vi "Fit parameters chooser.vi"(0 "Stop signaller":refnum<class "Signaller.lvclass">, 5 "Fit parameters refnum":refnum<vi>, 7 "C refnum":refnum<vi>, 9 "Physical constants refnum":refnum<vi>, 11 "Simulation parameters semaphore":T1) -> ()   [LabVIEW 2015]
uses:
  Fit Parameters.ctl
  Physical Constants.ctl
  Motor controller/Signaller/Signaller.lvclass
  <vilib>/gmath/statdist.llb/Continuous PDF.vi
  <vilib>/gmath/statdist.llb/Normal PDF.vi
  <vilib>/gmath/NI_Gmath.lvlib
  <vilib>/Utility/config.llb/NI_LVConfig.lvlib
panel:
  in  "Overwrite selected preset":bool
  in  "Save as new preset":bool
  in  "Load from preset":bool
  in  "Choose preset":u16(ring) items=["Experimental data", "Test"]
  in  "Refresh graphs":bool
  in  "Update simulation parameters":bool
  in  "Physical constants":T2={"T1e (s)"=0.03, "T1n (s)"=1500.0}
  in  "C":dbl=0.000136073
  in  "Fit parameters":T3={"A"=0.572086, "S"=0.0835606, "M1"=140.286, "M2"=140.486}
  out "Steady state distribution":cluster{dbl[], dbl[]}(graph)
  out "Alpha/beta distributions":cluster{dbl[], dbl[]}[](graph)
  # "Explanation of fit parameters:\nThe parameters A, S, M1, and M2 control the distribution of alpha and beta as shown above. The steady state distribution will be computed from these.\nA: the height of the Gaussian distributions for alpha and beta\nS: the standard deviation of the Gaussian distributions for alpha and beta\nM1: the mean of the Gaussian distribution for beta\nM2: the mean of the Gaussian distribution for alpha"
  # "Internal controls"
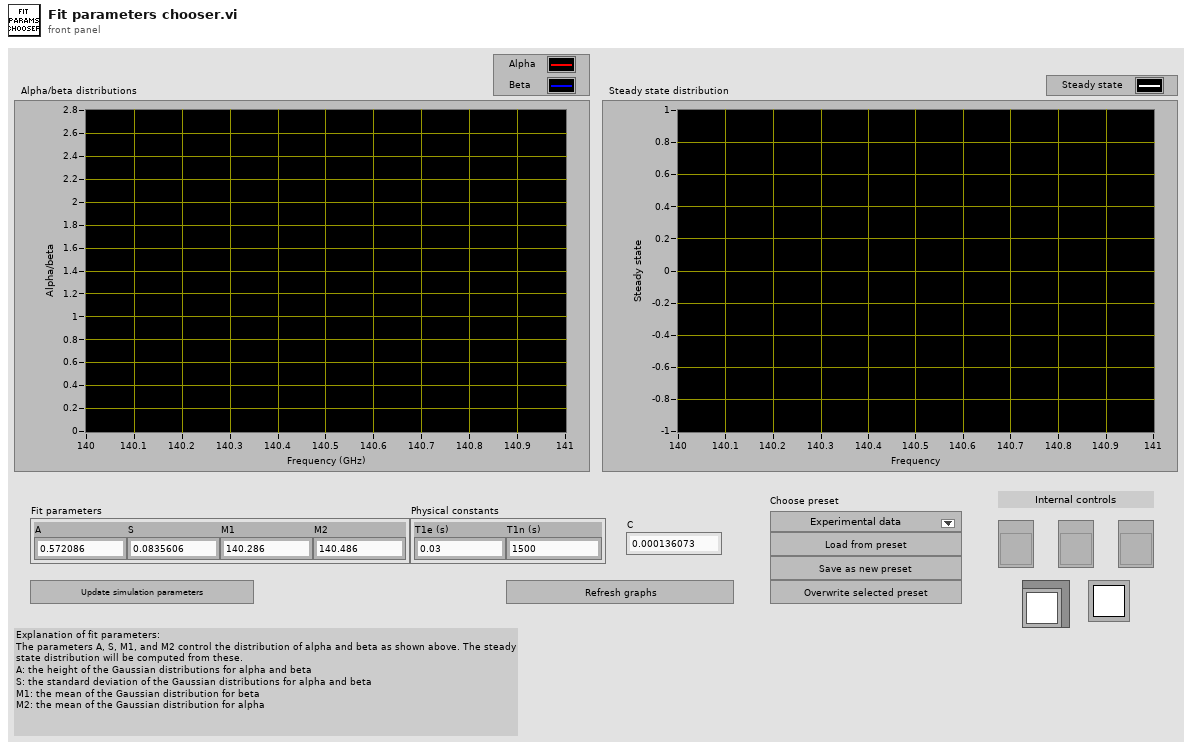
[diagram p1: front panel]
types:
  T1 = typedef "Semaphore RefNum" = refnum<k1>
  T2 = typedef "Physical Constants.ctl" = cluster{"T1e (s)":dbl, "T1n (s)":dbl}
  T3 = typedef "Fit Parameters.ctl" = cluster{"A":dbl, "S":dbl, "M1":dbl, "M2":dbl}
  T4 = typedef "LVRangeTypeDef.ctl" = cluster{"Minimum":dbl, "Maximum":dbl, "Increment":dbl, "Minor Increment":dbl, "Start":dbl}
  T5 = enum8{"Enabled", "Disabled", "Disabled and Grayed Out"}
  T6 = typedef "fit_parameters.ctl" = cluster{"A":dbl, "S":dbl, "M1":dbl, "M2":dbl}
  T7 = typedef "physical_constants.ctl" = cluster{"T1e (s)":dbl, "T1n (s)":dbl}
  T8 = typedef "NI_LVConfig.lvlib/Config Data RefNum.ctl" = refnum<k1>
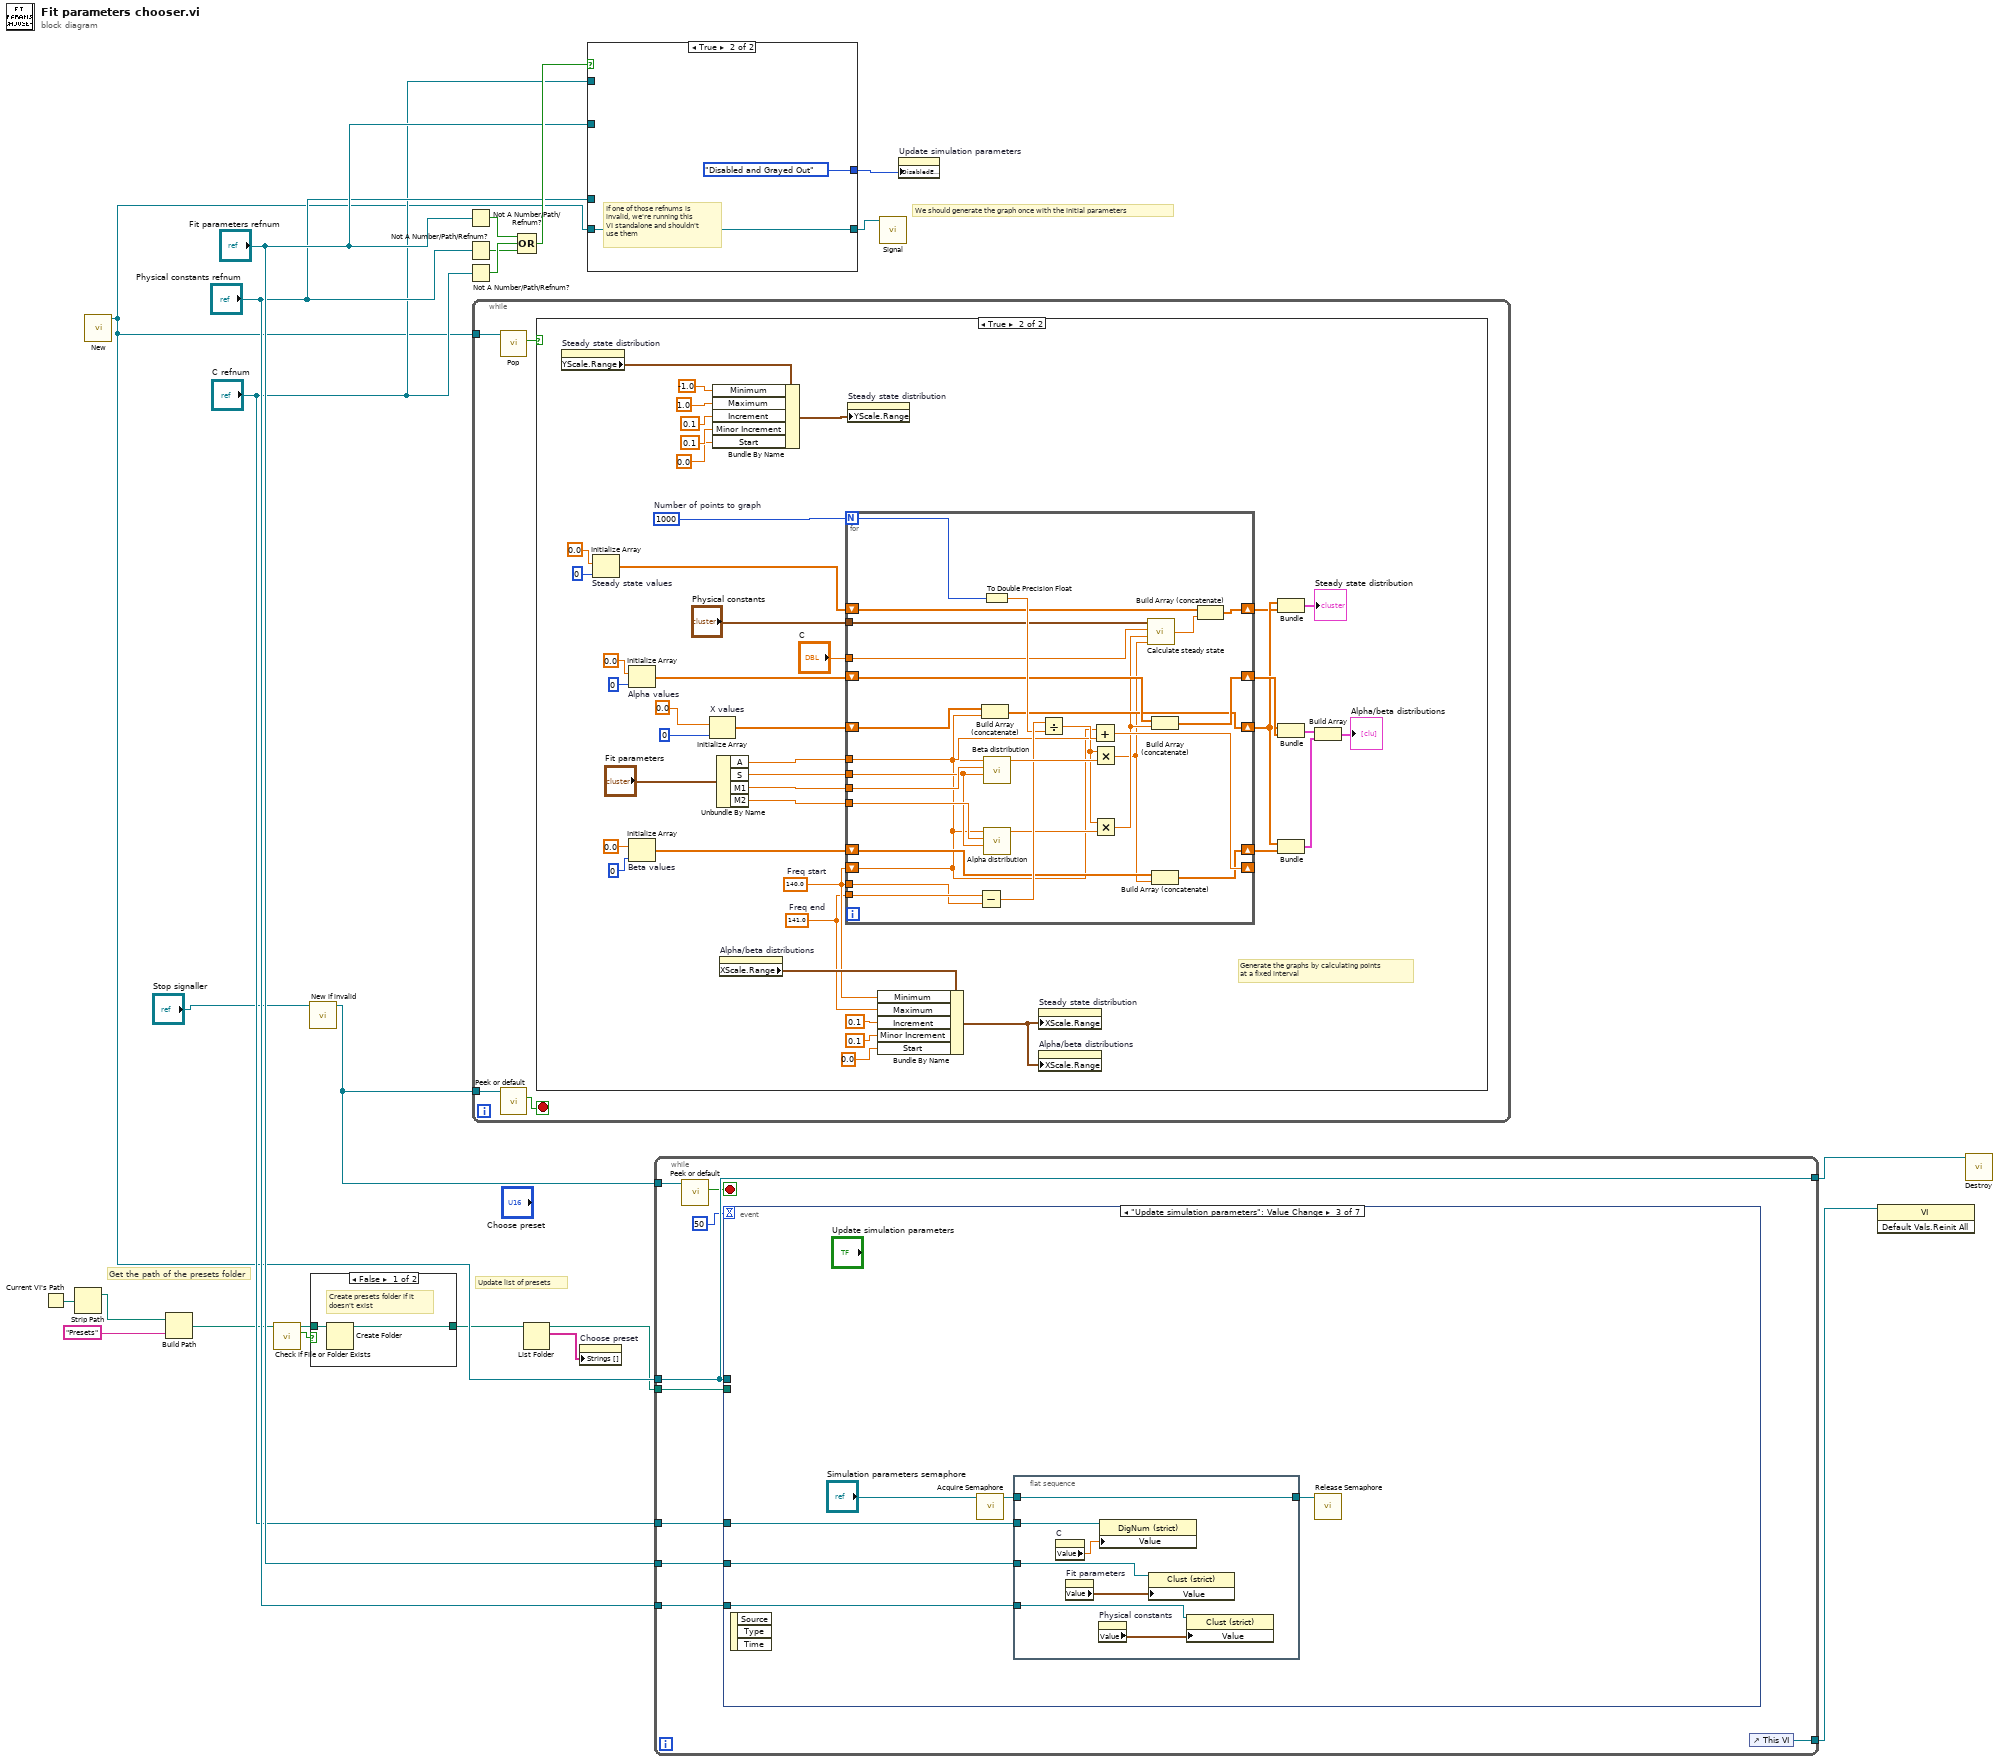
[diagram p0: block diagram]
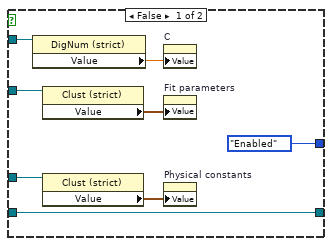
[diagram p3: hidden frame]
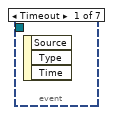
[diagram p4: hidden frame]
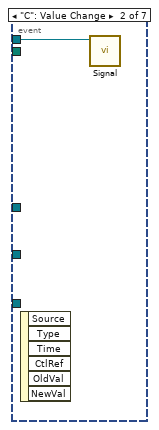
[diagram p5: hidden frame]
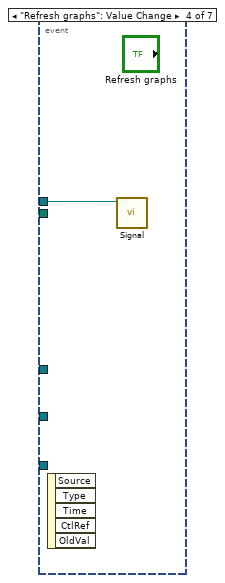
[diagram p6: hidden frame]
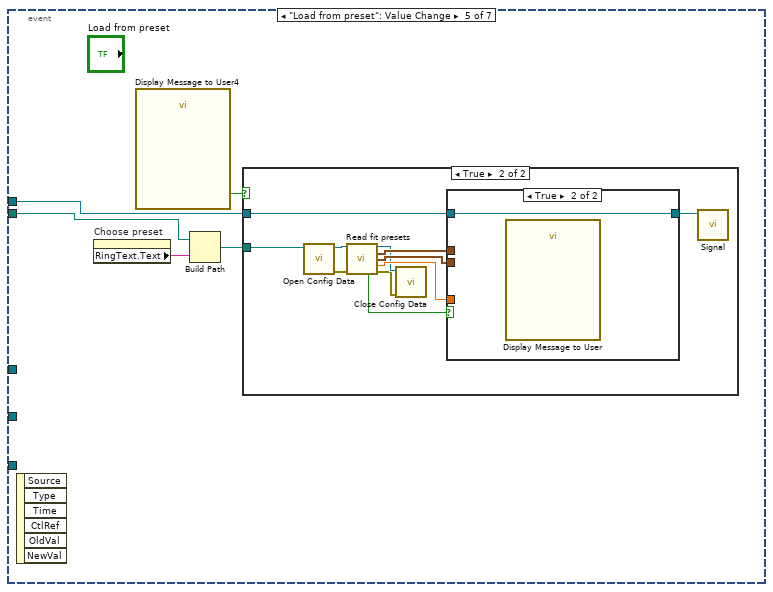
[diagram p7: hidden frame]
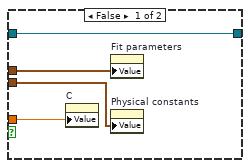
[diagram p9: hidden frame]
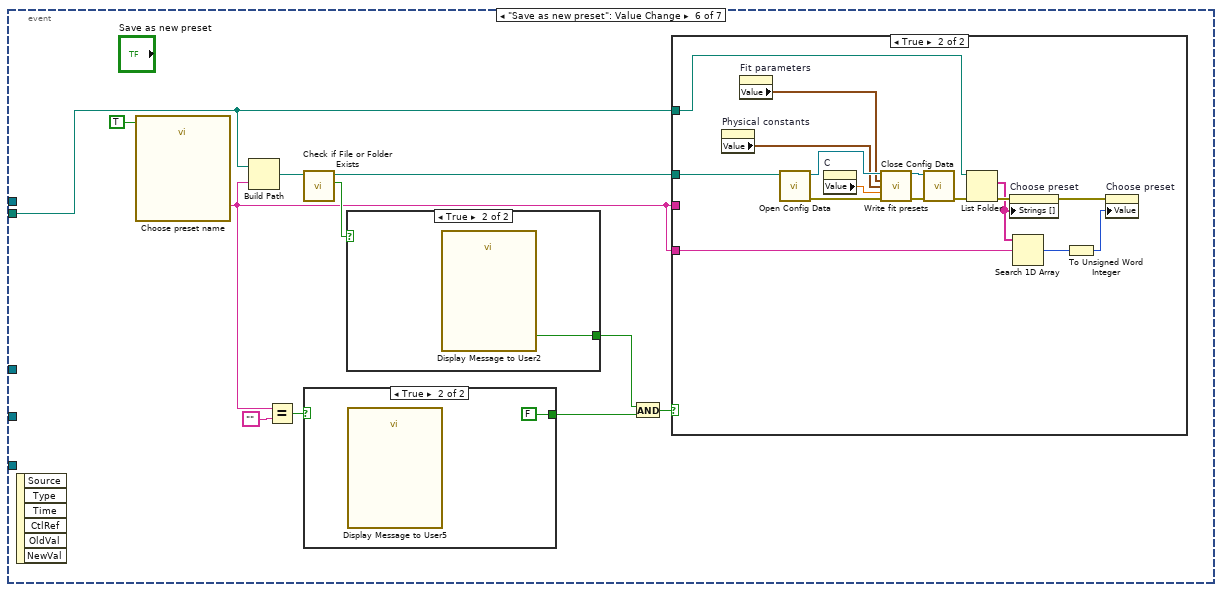
[diagram p10: hidden frame]
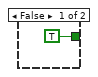
[diagram p11: hidden frame]
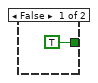
[diagram p13: hidden frame]
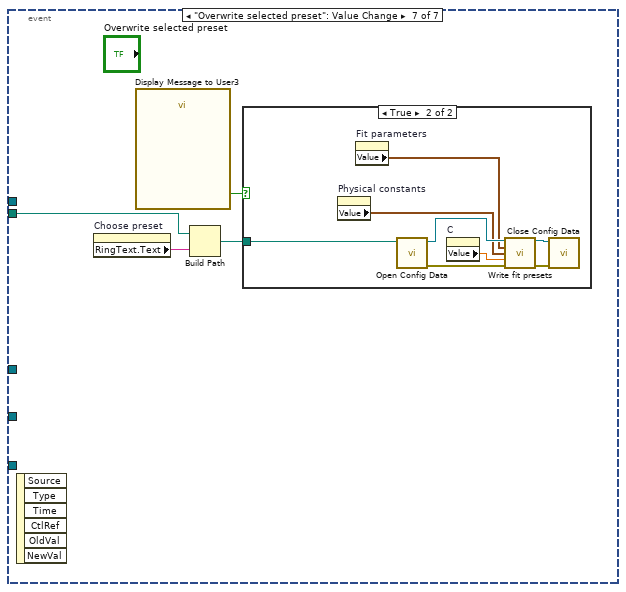
[diagram p14: hidden frame]
diagram:
  # "Update list of presets"
  # "Get the path of the presets folder"
  # "We should generate the graph once with the initial parameters"
  n1 = Current VI's Path() -> (path=w8:path)
  n2 = Strip Path(path=w8) -> (stripped path=w9:path)  [unwired: 1 out]
  n3 = call "New.vi"() -> ("Signaller out"=w12:refnum<class "Signaller.lvclass">)  [unwired: 11 in]
  n4 = Build Path(base path=w9, name or relative path="Presets") -> (appended path=w7:path)
  n5 = call <vilib>:"Check if File or Folder Exists.vi"("path"=w7) -> ("file or folder exists?"=w6:bool, "dup path"=w5:path)  [unwired: 8 in, 1 out]
  n6 = call "New if invalid.vi"("Signaller in"="Stop signaller") -> ("Signaller out"=w11:refnum<class "Signaller.lvclass">)  [unwired: 9 in, 1 out]
  n7 = case shown="False" w6 {
    tunnel: w5 -> [w25 w26]
    tunnel: [w24 w26] -> w4
    frame False {
      # "Create presets folder if it\ndoesn't exist"
      n8 = Create Folder(path (use dialog)=w25) -> (created path=w24:path)  [unwired: 2 in, 2 out]
    }
    frame True {
    }
  }
  n9 = Not A Number/Path/Refnum?(number/path/refnum="Fit parameters refnum") -> (NaN/Path/Refnum?=w21:bool)
  n10 = Not A Number/Path/Refnum?(number/path/refnum="Physical constants refnum") -> (NaN/Path/Refnum?=w19:bool)
  n11 = Not A Number/Path/Refnum?(number/path/refnum="C refnum") -> (NaN/Path/Refnum?=w20:bool)
  n12 = while {
    tunnel: w12 -> [w29]
    tunnel: w11 -> [w28]
    stop <- w27 stop-if-true
    n13 = call "Pop.vi"("Signaller in"=w29) -> ("Has signal"=w30:bool)  [unwired: 8 in, 2 out]
    n14 = call "Peek or default.vi"("Signaller in"=w28) -> ("Has signal?"=w27:bool)  [unwired: 8 in, 2 out]
    n15 = case shown="True" w30 {
      frame False {
      }
      frame True {
        w65 = 141.0  # Freq end
        w66 = 140.0  # Freq start
        w71 = 1000  # Number of points to graph
        # "Generate the graphs by calculating points\nat a fixed interval"
        n16 = property on="Steady state distribution" class="XYGraph (strict)"() -> ("YScale.Range"=w37:T4)  [unwired: 2 in, 2 out]
        n17 = Initialize Array "Steady state values"(0.0 ("element"), 0 ("dimension size")) -> (w43:dbl[])
        n18 = Initialize Array "Alpha values"(0.0 ("element"), 0 ("dimension size")) -> (w52:dbl[])
        n19 = Initialize Array "Beta values"(0.0 ("element"), 0 ("dimension size")) -> (w53:dbl[])
        n20 = Initialize Array "X values"(0.0 ("element"), 0 ("dimension size")) -> (w58:dbl[])
        n21 = Bundle By Name(cluster=w37, "Minimum"=-1.0, "Maximum"=1.0, "Increment"=0.1, "Minor Increment"=0.1, "Start"=0.0) -> (w36:T4)
        n22 = Unbundle By Name("Fit parameters") -> ("A"=w70:dbl, "S"=w68:dbl, "M1"=w69:dbl, "M2"=w61:dbl)
        n23 = property on="Alpha/beta distributions" class="XYGraph (strict)"() -> ("XScale.Range"=w67:T4)  [unwired: 2 in, 2 out]
        n24 = for {
          N: w71 -> [w93]
          shift-right: [w91] -> _
          shift-left: w66 -> [w80]
          tunnel: w70 -> [w84]
          tunnel: w69 -> [w98]
          tunnel: w68 -> [w89]
          tunnel: w65 -> [w97]
          tunnel: w66 -> [w96]
          tunnel: w61 -> [w90]
          shift-right: [w81] -> w42
          shift-left: w58 -> [w88]
          shift-right: [w83] -> w50
          shift-left: w53 -> [w86]
          shift-right: [w82] -> w51
          shift-left: w52 -> [w87]
          shift-right: [w77] -> w41
          shift-left: w43 -> [w79]
          tunnel: "Physical constants" -> [w76]
          tunnel: "C" -> [w75]
          n25 = Subtract(x=w97, y=w96) -> (x-y=w95:dbl)
          n26 = Build Array (concatenate)(w88, w80) -> (w81:dbl[])
          n27 = To Double Precision Float(number=w93) -> (double precision float=w94:dbl)
          n28 = call-poly "Beta distribution"("std"=w89, "mean"=w98, "x"=w80) -> ("pdf(x)"=w99:dbl)  [unwired: 7 in, 1 out]
          n29 = call-poly "Alpha distribution"("std"=w89, "mean"=w90, "x"=w80) -> ("pdf(x)"=w85:dbl)  [unwired: 7 in, 1 out]
          n30 = Divide(x=w95, y=w94) -> (x/y=w92:dbl)
          n31 = Add(x=w80, y=w92) -> (x+y=w91:dbl)
          n32 = Multiply(x=w84, y=w99) -> (x*y=w73:dbl)
          n33 = Multiply(x=w84, y=w85) -> (x*y=w74:dbl)
          n34 = call "Calculate steady state.vi"("Beta"=w73, "Alpha"=w74, "C"=w75, "Physical constants"=w76) -> ("Steady state"=w78:dbl)
          n35 = Build Array (concatenate)(w87, w74) -> (w82:dbl[])
          n36 = Build Array (concatenate)(w86, w73) -> (w83:dbl[])
          n37 = Build Array (concatenate)(w79, w78) -> (w77:dbl[])
        }
        n38 = property on="Steady state distribution" class="XYGraph (strict)"("YScale.Range"=w36) -> ()  [unwired: 2 in, 2 out]
        n39 = Bundle By Name(cluster=w67, "Minimum"=w66, "Maximum"=w65, "Increment"=0.1, "Minor Increment"=0.1, "Start"=0.0) -> (w46:T4)
        n40 = property on="Steady state distribution" class="XYGraph (strict)"("XScale.Range"=w46) -> ()  [unwired: 2 in, 2 out]
        n41 = property on="Alpha/beta distributions" class="XYGraph (strict)"("XScale.Range"=w46) -> ()  [unwired: 2 in, 2 out]
        n42 = Bundle(w42, w41) -> (→"Steady state distribution":cluster{dbl[], dbl[]})  [unwired: 1 in]
        n43 = Bundle(w42, w51) -> (w49:cluster{dbl[], dbl[]})  [unwired: 1 in]
        n44 = Bundle(w42, w50) -> (w48:cluster{dbl[], dbl[]})  [unwired: 1 in]
        n45 = Build Array(w49, w48) -> (→"Alpha/beta distributions":cluster{dbl[], dbl[]}[])
      }
    }
  }
  n46 = Compound Arithmetic op=OR(w21, w20, w19) -> (w22:bool)
  n47 = List Folder(path=w4) -> (path out=w2:path, filenames=w3:string[])  [unwired: 3 in, 2 out]
  n48 = property on="Choose preset" class="Ring (strict)"("Strings []"=w3) -> ()  [unwired: 2 in, 2 out]
  n49 = case shown="True" w22 {
    tunnel: [T5."Enabled" ("Disabled") T5."Disabled and Grayed Out" ("Disabled")] -> w18
    tunnel: "Fit parameters refnum" -> [w106 _]
    tunnel: "C refnum" -> [w104 _]
    tunnel: "Physical constants refnum" -> [w103 _]
    tunnel: w12 -> [w100 w108]
    tunnel: [w100 w108] -> w17
    frame False {
      n50 = property class="DigNum (strict)"(reference=w104) -> ("Value"=w102:dbl)  [unwired: 1 in, 2 out]
      n51 = property class="Clust (strict)"(reference=w106) -> ("Value"=w105:T6)  [unwired: 1 in, 2 out]
      n52 = property class="Clust (strict)"(reference=w103) -> ("Value"=w101:T7)  [unwired: 1 in, 2 out]
      n53 = property on="C" class="DigNum (strict)"("Value"=w102) -> ()  [unwired: 2 in, 2 out]
      n54 = property on="Fit parameters" class="Clust (strict)"("Value"=w105) -> ()  [unwired: 2 in, 2 out]
      n55 = property on="Physical constants" class="Clust (strict)"("Value"=w101) -> ()  [unwired: 2 in, 2 out]
    }
    frame True {
      # "If one of those refnums is\ninvalid, we're running this\nVI standalone and shouldn't\nuse them"
    }
  }
  n56 = while {
    tunnel: w12 -> [w118]
    tunnel: [w118] -> w23
    tunnel: "Fit parameters refnum" -> [w117]
    tunnel: "Physical constants refnum" -> [w116]
    tunnel: "C refnum" -> [w115]
    tunnel: w11 -> [w113]
    tunnel: w2 -> [w111]
    tunnel: [w110] -> w1
    stop <- w114 stop-if-true
    n57 = call "Peek or default.vi"("Signaller in"=w113) -> ("Has signal?"=w114:bool)  [unwired: 8 in, 2 out]
    n58 = event shown="[2] \"Update simulation parameters\": Value Change" {
      selector: _ -> [_ _ _ _ _ _ _]
      dyn-events: _ -> [_ _ _ _ _ _ _]
      timeout: 50 -> [_ _ _ _ _ _ _]
      tunnel: w118 -> [_ w119 _ w133 w134 _ _]
      tunnel: w117 -> [_ _ w125 _ _ _ _]
      tunnel: w116 -> [_ _ w124 _ _ _ _]
      tunnel: w115 -> [_ _ w123 _ _ _ _]
      tunnel: w111 -> [_ _ _ _ w138 w162 w189]
      event Timeout {
        n59 = event-data() -> ()  [unwired: 1 in, 3 out]
      }
      event "C": Value Change {
        n60 = event-data() -> ()  [unwired: 1 in, 6 out]
        n61 = call "Signal.vi"("Signaller in"=w119) -> ()  [unwired: 9 in, 2 out]
      }
      event "Update simulation parameters": Value Change {
        n62 = event-data() -> ()  [unwired: 1 in, 3 out]
        n63 = call <vilib>:"Acquire Semaphore.vi"("semaphore"="Simulation parameters semaphore") -> ("semaphore out"=w121:T1)  [unwired: 4 in, 2 out]
        n64 = flat-sequence {
          tunnel: w125 -> [w132]
          tunnel: w124 -> [w131]
          tunnel: w123 -> [w130]
          tunnel: w121 -> [w126]
          tunnel: [w126] -> w120
          frame #0 {
            n65 = property on="C" class="DigNum (strict)"() -> ("Value"=w127:dbl)  [unwired: 2 in, 2 out]
            n66 = property on="Fit parameters" class="Clust (strict)"() -> ("Value"=w129:T6)  [unwired: 2 in, 2 out]
            n67 = property on="Physical constants" class="Clust (strict)"() -> ("Value"=w128:T7)  [unwired: 2 in, 2 out]
            n68 = property class="DigNum (strict)"(reference=w130, "Value"=w127) -> ()  [unwired: 1 in, 2 out]
            n69 = property class="Clust (strict)"(reference=w132, "Value"=w129) -> ()  [unwired: 1 in, 2 out]
            n70 = property class="Clust (strict)"(reference=w131, "Value"=w128) -> ()  [unwired: 1 in, 2 out]
          }
        }
        n71 = call <vilib>:"Release Semaphore.vi"("semaphore"=w120) -> ()  [unwired: 5 in, 2 out]
      }
      event "Refresh graphs": Value Change {
        n72 = event-data() -> ()  [unwired: 1 in, 5 out]
        n73 = call "Signal.vi"("Signaller in"=w133) -> ()  [unwired: 9 in, 2 out]
      }
      event "Load from preset": Value Change {
        n74 = event-data() -> ()  [unwired: 1 in, 6 out]
        n75 = property on="Choose preset" class="Ring (strict)"() -> ("RingText.Text"=w137:string)  [unwired: 2 in, 2 out]
        n76 = call "Display Message to User4"() -> ("Yes"=w135:bool)  [unwired: 10 in, 1 out]
        n77 = Build Path(base path=w138, name or relative path=w137) -> (appended path=w136:path)
        n78 = case shown="True" w135 {
          tunnel: w136 -> [_ w149]
          tunnel: w134 -> [_ w140]
          frame False {
          }
          frame True {
            n79 = call <vilib>:"Open Config Data.vi"("configuration file path"=w149) -> ("error out"=w142:errorcluster, "refnum"=w148:T8)  [unwired: 8 in, 1 out]
            n80 = call "Read fit presets.vi"("Config file in"=w148, "error in (no error)"=w142) -> ("Config file out"=w143:T8, "Fit parameters"=w147:T3, "Physical constants"=w146:T2, "C"=w145:dbl, "Key not found?"=w144:bool, "error out"=w141:errorcluster)  [unwired: 8 in]
            n81 = call <vilib>:"Close Config Data.vi"("error in (no error)"=w141, "refnum"=w143) -> ()  [unwired: 8 in, 2 out]
            n82 = case shown="True" w144 {
              tunnel: w147 -> [w153 _]
              tunnel: w146 -> [w152 _]
              tunnel: w145 -> [w151 _]
              tunnel: w140 -> [w150 w154]
              tunnel: [w150 w154] -> w139
              frame False {
                n83 = property on="C" class="DigNum (strict)"("Value"=w151) -> ()  [unwired: 2 in, 2 out]
                n84 = property on="Fit parameters" class="Clust (strict)"("Value"=w153) -> ()  [unwired: 2 in, 2 out]
                n85 = property on="Physical constants" class="Clust (strict)"("Value"=w152) -> ()  [unwired: 2 in, 2 out]
              }
              frame True {
                n86 = call "Display Message to User"() -> ()  [unwired: 10 in, 2 out]
              }
            }
            n87 = call "Signal.vi"("Signaller in"=w139) -> ()  [unwired: 9 in, 2 out]
          }
        }
      }
      event "Save as new preset": Value Change {
        n88 = event-data() -> ()  [unwired: 1 in, 6 out]
        n89 = call "Choose preset name"("Enable"=TRUE) -> ("Preset name"=w159:string)  [unwired: 16 in, 2 out]
        n90 = Build Path(base path=w162, name or relative path=w159) -> (appended path=w165:path)
        n91 = Equal?(x=w159, y="") -> (x = y?=w158:bool)
        n92 = call <vilib>:"Check if File or Folder Exists.vi"("path"=w165) -> ("file or folder exists?"=w164:bool, "dup path"=w163:path)  [unwired: 8 in, 1 out]
        n93 = case shown="True" w158 {
          tunnel: [TRUE FALSE] -> w155
          frame False {
          }
          frame True {
            n94 = call "Display Message to User5"() -> ()  [unwired: 10 in, 2 out]
          }
        }
        n95 = case shown="True" w164 {
          tunnel: [TRUE ("Yes") w185] -> w156
          frame False {
          }
          frame True {
            n96 = call "Display Message to User2"() -> ("Yes"=w185:bool)  [unwired: 10 in, 1 out]
          }
        }
        n97 = And(x=w156, y=w155) -> (x .and. y?=w157:bool)
        n98 = case shown="True" w157 {
          tunnel: w163 -> [_ w183]
          tunnel: w159 -> [_ _]
          tunnel: w162 -> [_ w177]
          tunnel: w159 -> [_ w171]
          frame False {
          }
          frame True {
            n99 = property on="Physical constants" class="Clust (strict)"() -> ("Value"=w180:T7)  [unwired: 2 in, 2 out]
            n100 = property on="Fit parameters" class="Clust (strict)"() -> ("Value"=w181:T6)  [unwired: 2 in, 2 out]
            n101 = call <vilib>:"Open Config Data.vi"("configuration file path"=w183) -> ("error out"=w175:errorcluster, "refnum"=w182:T8)  [unwired: 8 in, 1 out]
            n102 = property on="C" class="DigNum (strict)"() -> ("Value"=w179:dbl)  [unwired: 2 in, 2 out]
            n103 = call "Write fit presets.vi"("Config file in"=w182, "Fit parameters"=w181, "Physical constants"=w180, "C"=w179, "error in (no error)"=w175) -> ("Config file out"=w178:T8, "error out"=w174:errorcluster)  [unwired: 9 in]
            n104 = call <vilib>:"Close Config Data.vi"("error in (no error)"=w174, "refnum"=w178) -> ("error out"=w176:errorcluster)  [unwired: 8 in, 1 out]
            n105 = List Folder(path=w177, error in=w176) -> (filenames=w172:string[], error out=w173:errorcluster)  [unwired: 2 in, 2 out]
            n106 = property on="Choose preset" class="Ring (strict)"(error in=w173, "Strings []"=w172) -> (error out=w168:errorcluster)  [unwired: 1 in, 1 out]
            n107 = Search 1D Array(1D array=w172, element=w171) -> (index of element=w170:i32)  [unwired: 1 in]
            n108 = To Unsigned Word Integer(number=w170) -> (unsigned 16bit integer=w169:u16)
            n109 = property on="Choose preset" class="Ring (strict)"(error in=w168, "Value"=w169) -> ()  [unwired: 1 in, 2 out]
          }
        }
      }
      event "Overwrite selected preset": Value Change {
        n110 = event-data() -> ()  [unwired: 1 in, 6 out]
        n111 = property on="Choose preset" class="Ring (strict)"() -> ("RingText.Text"=w188:string)  [unwired: 2 in, 2 out]
        n112 = call "Display Message to User3"() -> ("Yes"=w187:bool)  [unwired: 10 in, 1 out]
        n113 = Build Path(base path=w189, name or relative path=w188) -> (appended path=w186:path)
        n114 = case shown="True" w187 {
          tunnel: w186 -> [_ w197]
          frame False {
          }
          frame True {
            n115 = property on="Physical constants" class="Clust (strict)"() -> ("Value"=w194:T7)  [unwired: 2 in, 2 out]
            n116 = property on="Fit parameters" class="Clust (strict)"() -> ("Value"=w195:T6)  [unwired: 2 in, 2 out]
            n117 = call <vilib>:"Open Config Data.vi"("configuration file path"=w197) -> ("error out"=w191:errorcluster, "refnum"=w196:T8)  [unwired: 8 in, 1 out]
            n118 = property on="C" class="DigNum (strict)"() -> ("Value"=w193:dbl)  [unwired: 2 in, 2 out]
            n119 = call "Write fit presets.vi"("Config file in"=w196, "Fit parameters"=w195, "Physical constants"=w194, "C"=w193, "error in (no error)"=w191) -> ("Config file out"=w192:T8, "error out"=w190:errorcluster)  [unwired: 9 in]
            n120 = call <vilib>:"Close Config Data.vi"("error in (no error)"=w190, "refnum"=w192) -> ()  [unwired: 8 in, 2 out]
          }
        }
      }
    }
    n121 = control-ref of="This VI"() -> (w110:refnum<vi>)
  }
  n122 = call "Signal.vi"("Signaller in"=w17) -> ()  [unwired: 9 in, 2 out]
  n123 = property on="Update simulation parameters" class="Bool"("DisabledEnum"=w18) -> ()  [unwired: 2 in, 2 out]
  n124 = invoke class="VI" method="Default Vals.Reinit All"(reference=w1) -> ()  [unwired: 2 in, 3 out]
  n125 = call "Destroy.vi"("Signaller in"=w23) -> ()  [unwired: 10 in, 1 out]
